vi "On Change Take Calibration Sample.vi"(8 "error in (no error)":errorcluster, 10 "Value":bool, 11 "App in":refnum<class "App.lvclass">) -> (0 "error out":errorcluster, 3 "App out":refnum<class "App.lvclass">)   [LabVIEW 2020, in "AR Example.lvlib" / "App.lvclass"]
uses:
  App.lvclass
  App.lvclass/App.ctl
  UI/UI.lvclass
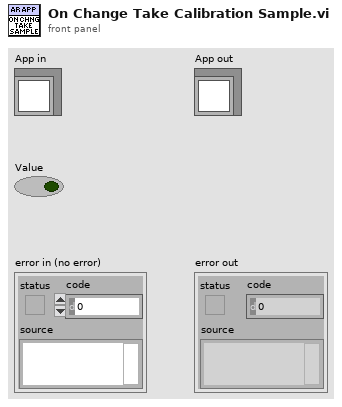
[diagram p1: front panel]
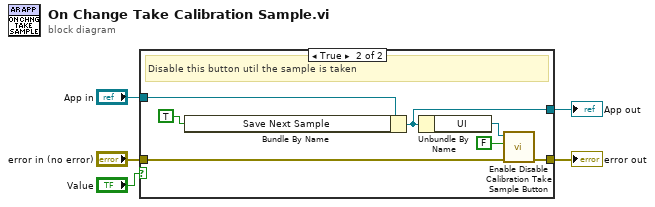
[diagram p0: block diagram]
diagram:
  n1 = case shown="True" "Value" {
    tunnel: "error in (no error)" -> [w6 w14]
    tunnel: "App in" -> [w7 w13]
    tunnel: [w7 w11] -> w3
    tunnel: [w6 w10] -> w2
    frame False {
    }
    frame True {
      # "Disable this button util the sample is taken"
      n2 = Bundle By Name(cluster=w13, "Save Next Sample"=TRUE ("Camera Calibration.Save Next Sample")) -> (w11:refnum<class "App.lvclass">)
      n3 = Unbundle By Name(w11) -> ("UI"=w9:refnum<class "UI.lvclass">)
      n4 = call-dynamic "Enable Disable Calibration Take Sample Button.vi"("error in (no error)"=w14, "Enable?"=FALSE, "UI in"=w9) -> ("error out"=w10:errorcluster)  [unwired: 8 in]
    }
  }
  "error out" <- w2
  "App out" <- w3
